vi "Unflatten-PenMotionEventData.vi"(8 "error in (no error)":errorcluster, 11 "Event Binary Data":string) -> (0 "error out":errorcluster, 3 "Event Data":T1 {"Pen State" items=["SDL_PEN_INPUT_DOWN"=1, "SDL_PEN_INPUT_BUTTON_1"=2, "SDL_PEN_INPUT_BUTTON_2"=4, "SDL_PEN_INPUT_BUTTON_3"=8, "SDL_PEN_INPUT_BUTTON_4"=16, "SDL_PEN_INPUT_BUTTON_5"=32, "SDL_PEN_INPUT_ERASER_TIP"=1073741824]})   [LabVIEW 2026, in "SDL3.lvlib" / "Events.lvlib"]
uses:
  PenMotionEventData--cluster.ctl
  Video/WindowID--integer.ctl
  Pen/PenID--integer.ctl
  Pen/PenInputFlags--ring.ctl
  Events.lvlib
  Video/Video.lvlib
  Pen/Pen.lvlib
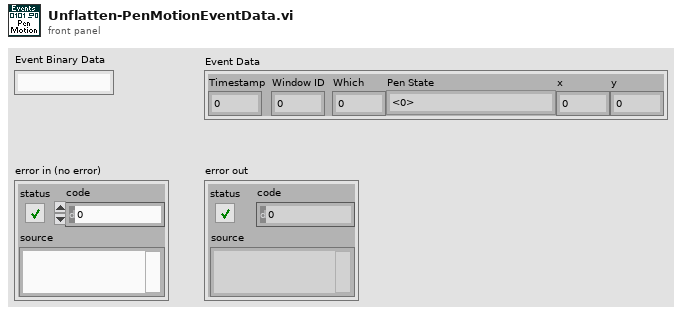
[diagram p1: front panel]
types:
  T1 = typedef "SDL3.lvlib/Events.lvlib/PenMotionEventData--cluster.ctl" = cluster{"Timestamp":u64, "Window ID":T2, "Which":T3, "Pen State":T4, "x":sgl, "y":sgl}
  T2 = typedef "SDL3.lvlib/Video.lvlib/WindowID--integer.ctl" = u32
  T3 = typedef "SDL3.lvlib/Pen.lvlib/PenID--integer.ctl" = u32
  T4 = typedef "SDL3.lvlib/Pen.lvlib/PenInputFlags--ring.ctl" = u32
  T5 = enum16{"big-endian, network order", "native, host order", "little-endian"}
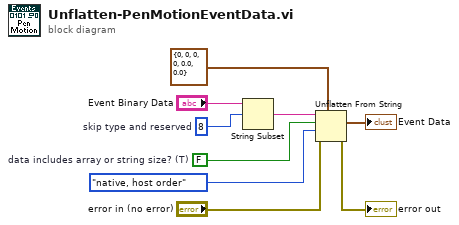
[diagram p0: block diagram]
diagram:
  w3 = 8  # skip type and reserved
  w6 = FALSE  # data includes array or string size? (T)
  n1 = String Subset(string="Event Binary Data", offset (0)=w3) -> (substring=w4:string)  [unwired: 1 in]
  n2 = Unflatten From String(type=T1 {"Timestamp"=0, "Window ID"=0, "Which"=0, "Pen State"=0, "x"=0.0, "y"=0.0} ("PenMotionEvent"), binary string=w4, data includes array or string size? (T)=w6, byte order (0:big-endian, network order)=T5."native, host order", error in (no error)="error in (no error)") -> (value=→"Event Data":T1, error out=→"error out":errorcluster)  [unwired: 1 out]
